vi "Count Num of True Element in 1D Array.vi"(8 "错误输入":errorcluster, 11 "Boolean Array(1D)":bool[](array[boolean])) -> (0 "错误输出":errorcluster, 3 "Num of True":i16)   [LabVIEW 2012]
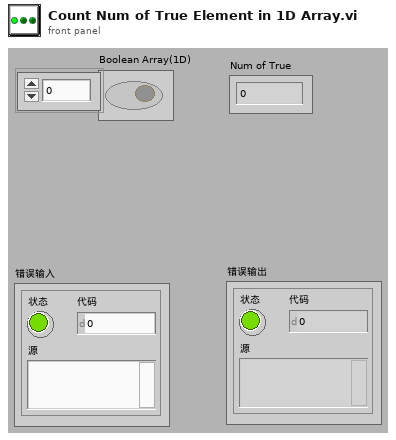
[diagram p1: front panel]
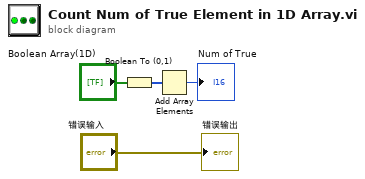
[diagram p0: block diagram]
diagram:
  n1 = Boolean To (0,1)(Boolean="Boolean Array(1D)") -> (0, 1=w4:i16[])
  n2 = Add Array Elements(numeric array=w4) -> (sum=→"Num of True":i16)
  "错误输出" <- "错误输入"
